vi "WDF file reader for YokaogawaDL850.vi"() -> ()   [LabVIEW 2010]
uses:
  <vilib>/Platform/storage/lvStorage.llb/xStorage/Open Data Storage/Open Data Storage.xnode
  <vilib>/Platform/storage/lvStorage.llb/_openFunction.ctl
  <vilib>/Platform/storage/lvStorage.llb/xStorage/Read Data/Read Data.xnode
  <vilib>/Platform/storage/lvStorage.llb/xStorage/Close Data Storage/Close Data Storage.xnode
  <vilib>/Analysis/3filter.llb/Filter Passband Type.ctl
  <vilib>/Platform/storage/lvStorage.llb/_openStorageWithRootAutoDetect.vi
  <vilib>/Platform/storage/lvStorage.llb/xStorage/xStorageSupp/ErrorOut.vi
  <vilib>/Platform/storage/lvStorage.llb/_queryPropDateTime.vi
  <vilib>/Platform/storage/lvStorage.llb/_queryGenericObjects.vi
  <vilib>/Platform/storage/lvStorage.llb/_loadAllDouble.vi
  <vilib>/Platform/storage/Storage.llb/Get Object Info.vi
  <vilib>/Platform/storage/Storage.llb/__closeStorageFromObject.vi
  <vilib>/Analysis/3filter.llb/Butterworth Filter (DBL).vi
  <vilib>/measure/maspectr.llb/FFT Power Spectrum and PSD for 1 Chan.vi
  <vilib>/Analysis/2dsp.llb/1D Auto Correlation (DBL).vi
  <vilib>/Analysis/2dsp.llb/1D Cross Correlation (DBL).vi
  <vilib>/Utility/file.llb/Write To Spreadsheet File (DBL).vi
  <vilib>/Utility/file.llb/Write To Spreadsheet File (string).vi
  <vilib>/measure/NI_MAPro.lvlib
  <vilib>/Analysis/NI_AALBase.lvlib
  <vilib>/Analysis/NI_AALPro.lvlib
panel:
  out "cross corr":dbl[](graph) caption="Rxx"
  in  "Check correlation":bool
  out "auto corr V":dbl[](graph) caption="Rxx"
  out "Rxx":dbl[](graph)
  in  "voltage Zero mean":bool
  in  "current Zero mean":bool
  out "saved selected data file name":string
  out "Moving average time":dbl
  in  "Moving average Window size":i32
  in  "Trace type":enum16{"current", "voltage"}(ring)
  in  "Check noise spectrum":bool
  out "Power spectrum":cluster{dbl[], "magnitude":dbl[]}(graph)
  out "Sampling rate (Hz)":dbl
  out "current trace":cluster{dbl[], "Data":dbl[]}(graph)
  in  "Save selected Data":bool
  in  "File type":string(combo)="*.wdf"
  in  "Save Data":bool
  in  "Voltage amplifier gain":dbl=10.0
  in  "Applied voltage(V)":dbl=0.1
  in  "Sampling interval (ms)":dbl=0.02
  out "CH-all":dbl[][](graph)
  out "Total data points":i32
  out "File Path":path=path "C:/JinHe/data/CNT measurement/20080324_SWCNT bundle/2MKCl1p2V5E40.txt"
  in  "Current No 2":u16
  in  "Forward":bool
  in  "back":bool
  in  "Change folder":bool
  in  "Current No":u16
  out "Total":dbl
  out "Status":string
  out "Numeric":i32
  in  "stop":bool
  out "error out":errorcluster
  out "Voltage trace":cluster{dbl[], "Array":dbl[]}[](graph)
  # "YOKOGAWA DL850 WDF file reader"
  # "Viewing files"
  # "(ms)"
  # "(points)"
  # "try save in TDMS format\nselect different noise removing function"
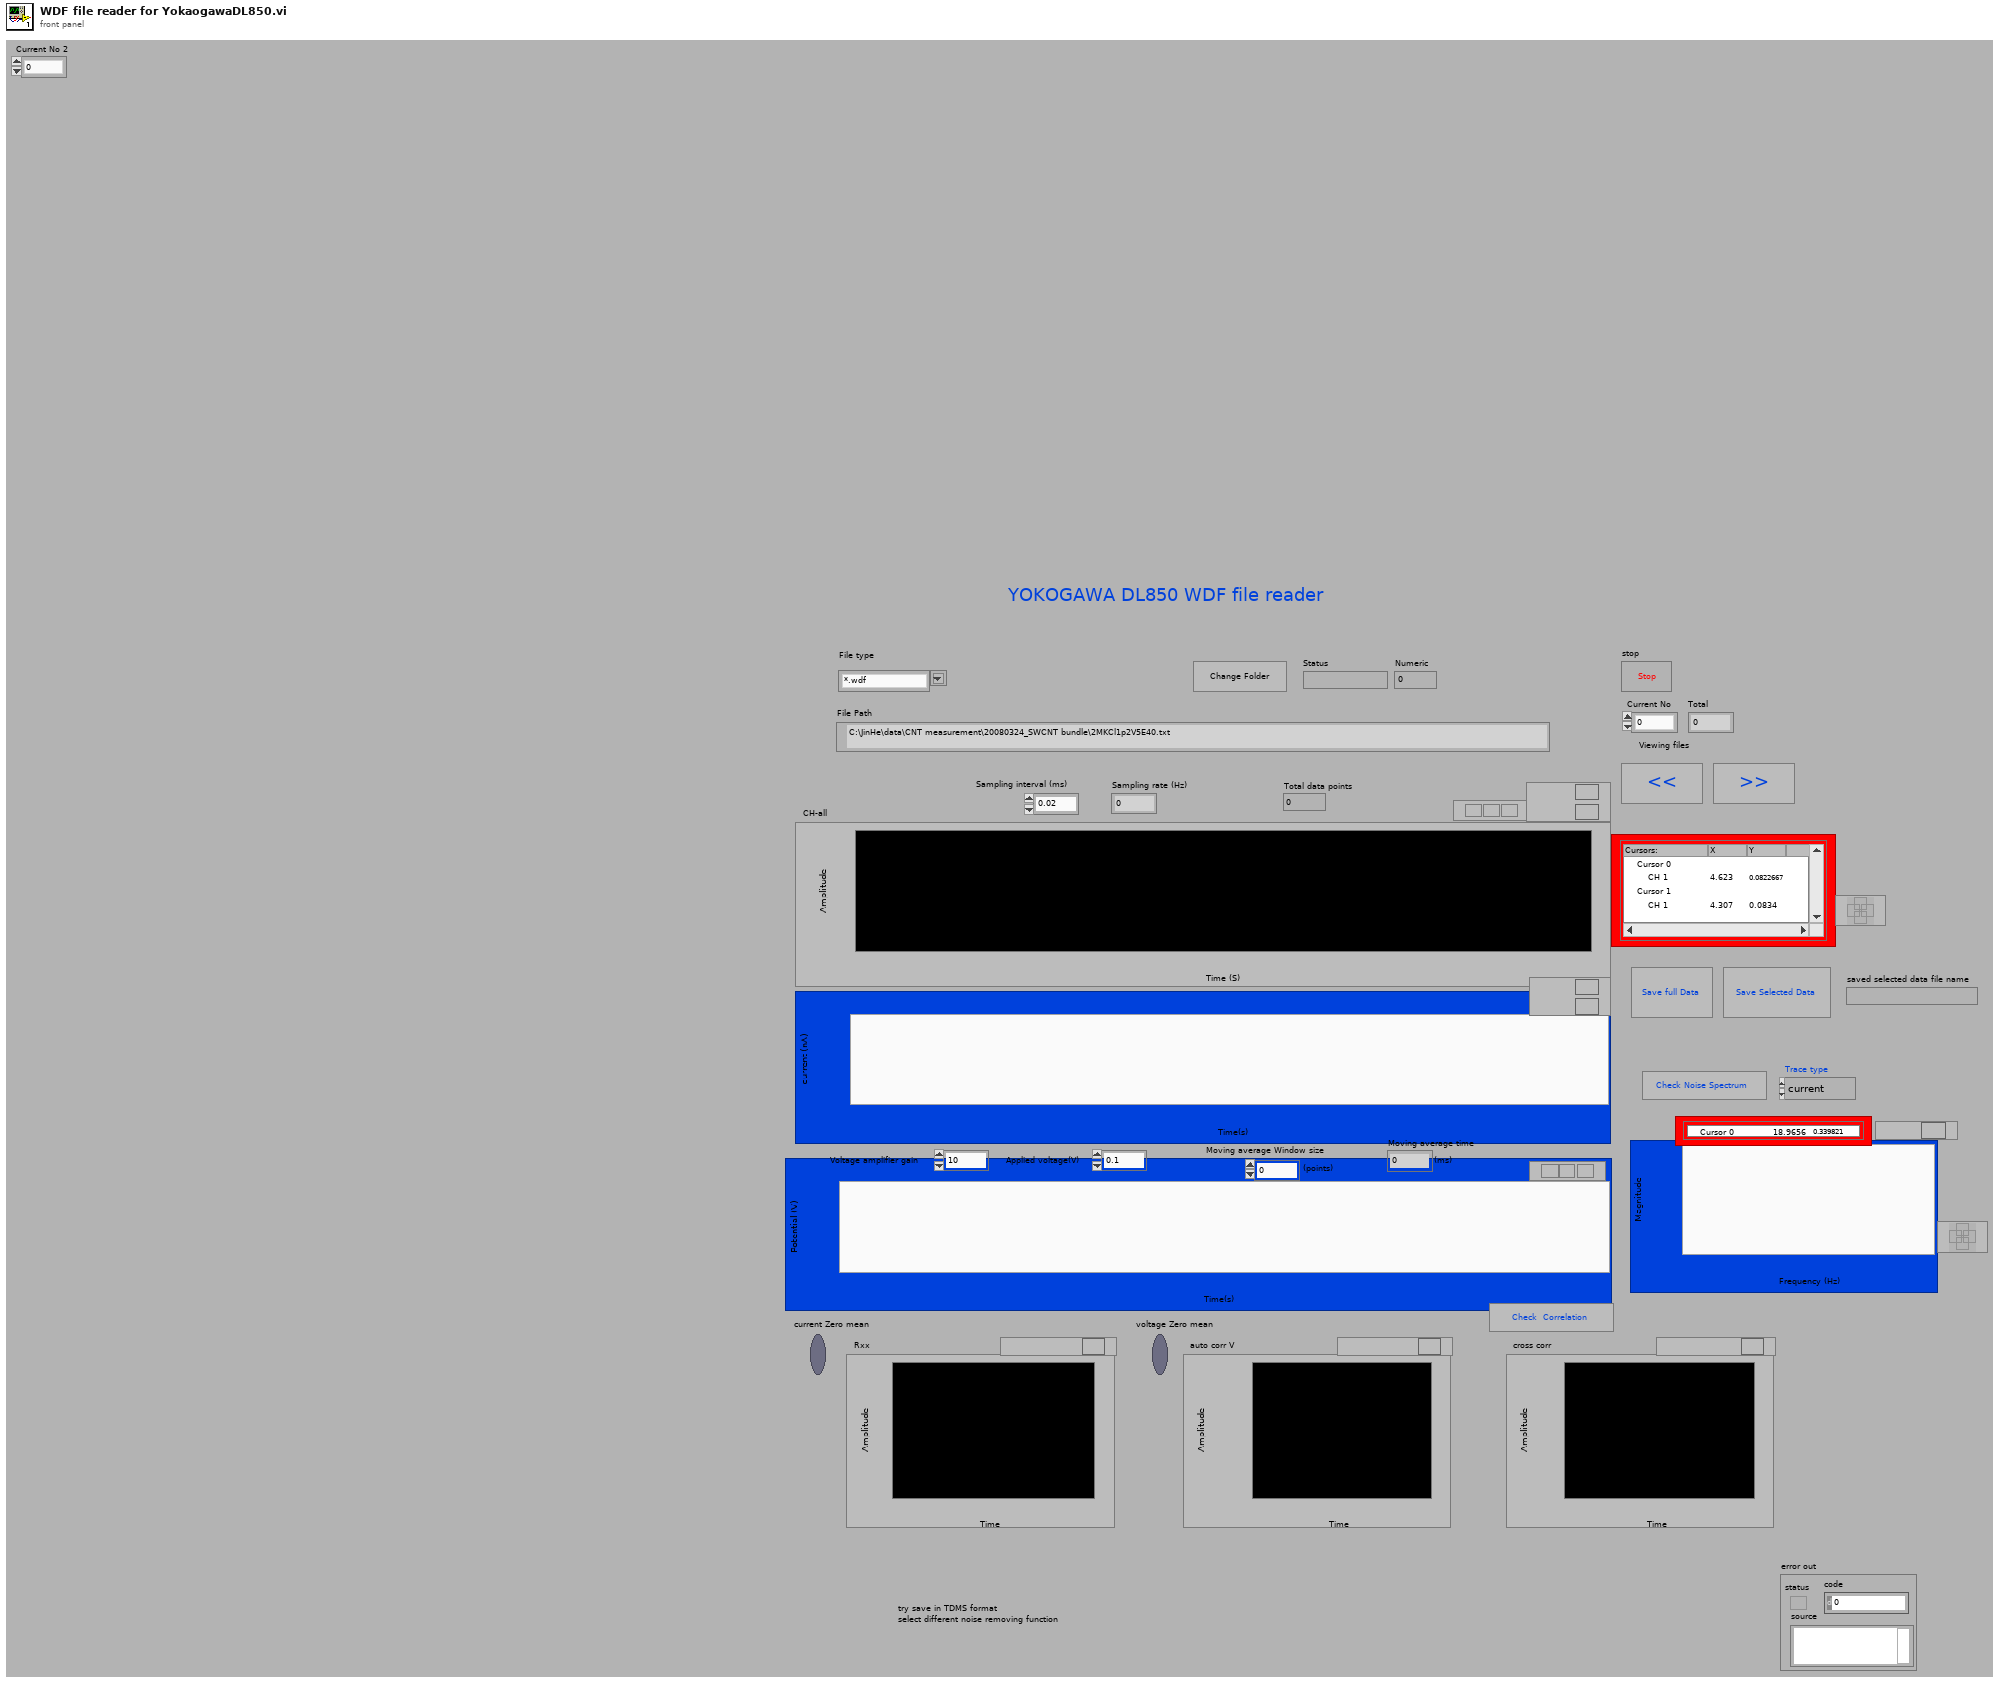
[diagram p1: front panel]
types:
  T1 = cluster{bool, "DIR path":path, "File names":string[], "File total number":i32, "File number counter":i32, "Data":dbl[][], "offset":dbl, "Peaks":dbl[][], "Step":dbl, "High":dbl, "Low":dbl, "Start":dbl, "End":dbl, "timestep(s)":dbl, "Modified Data ":dbl[][], "voltage gain":dbl, "Baseline":dbl[], "Magnitude":dbl[][], "Applied voltage (V)":dbl, "Data number":i32, "current data":dbl[][], "voltage data":dbl[][], "File type":string, "Cursor X1":dbl, "Cursor X0":dbl, "Time":dbl[], "Selected data":dbl[][]}
  T2 = enum16{"UPDATE", "READ", "QUERY", "CREATE CHILD", "CREATE", "CONNECT", "DISCONNECT"}
  T3 = typedef "_openFunction.ctl" = enum16{"open", "open or create", "create or replace", "create", "open (read only)"}
  T4 = typedef "NI_AALBase.lvlib/Filter Passband Type.ctl" = enum32{"Lowpass", "Highpass", "Bandpass", "Bandstop"}
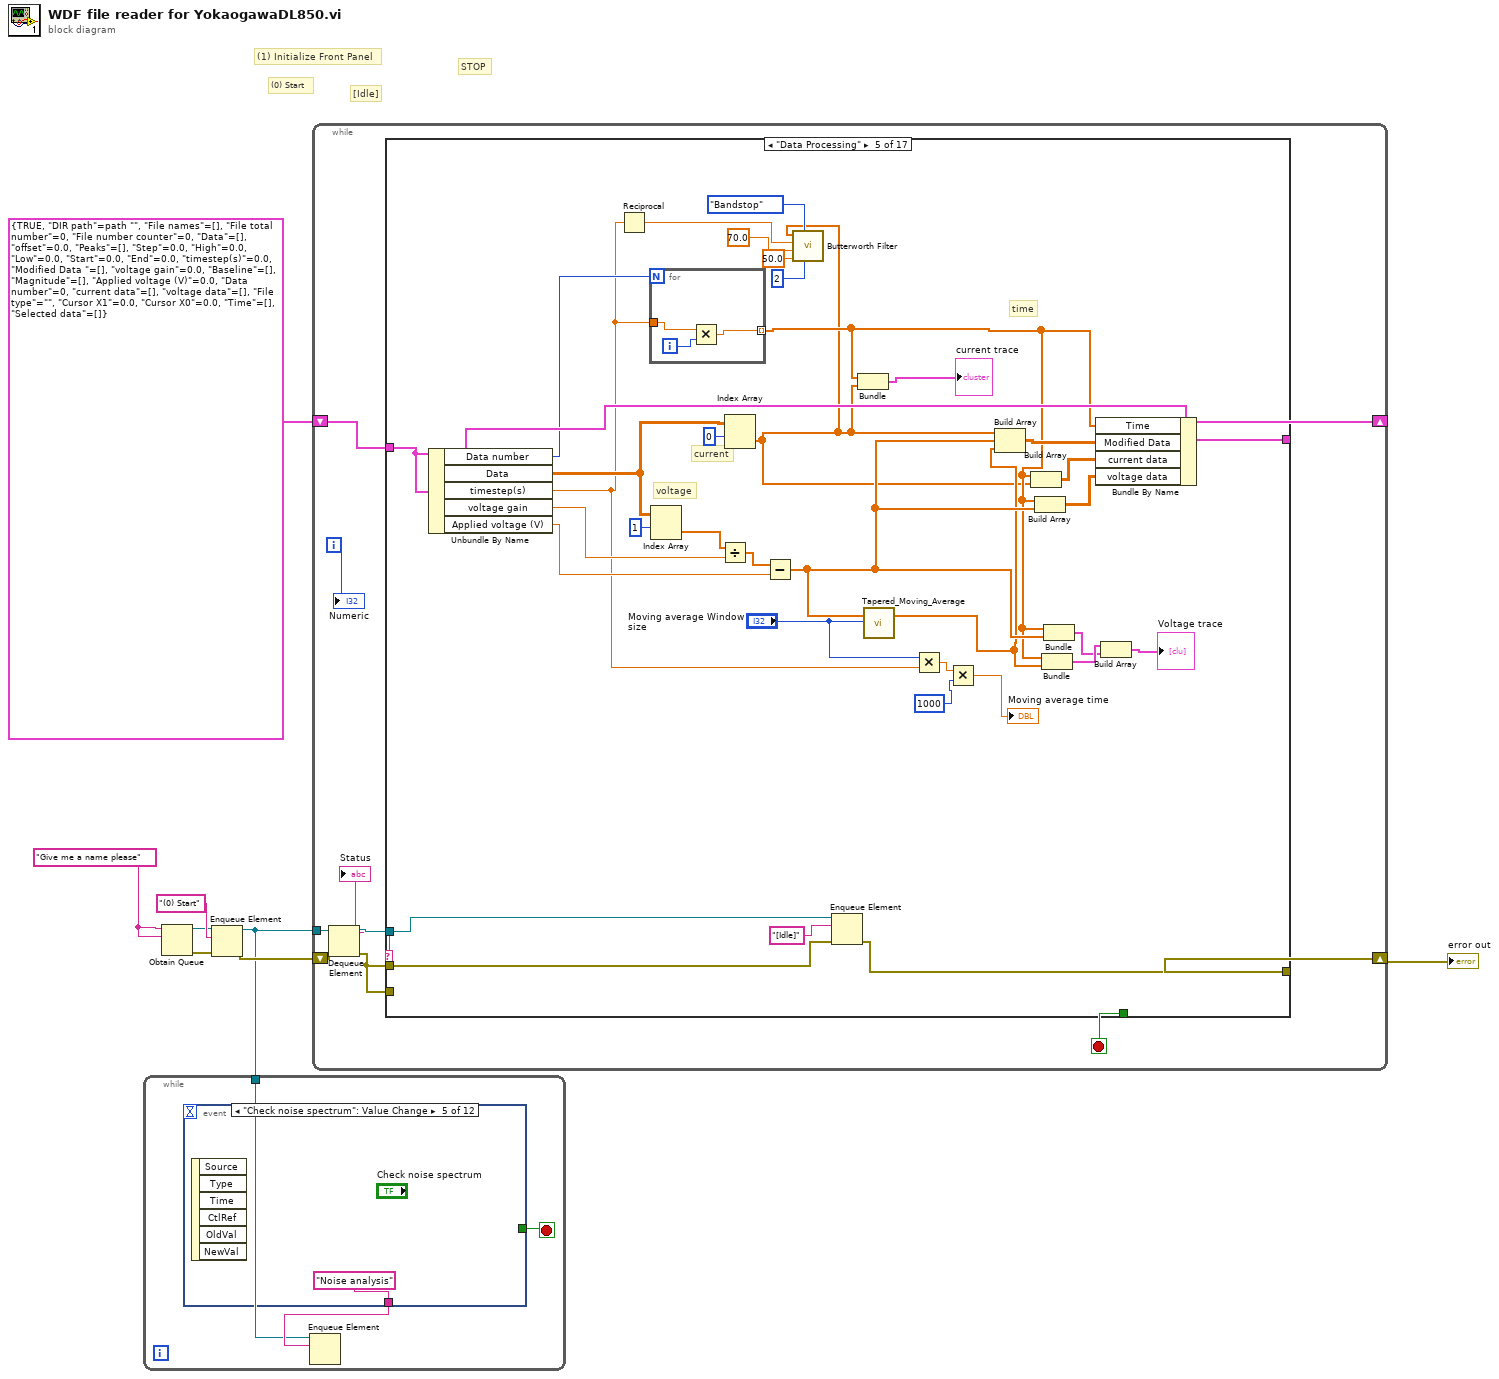
[diagram p0: block diagram]
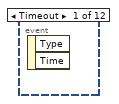
[diagram p2: hidden frame]
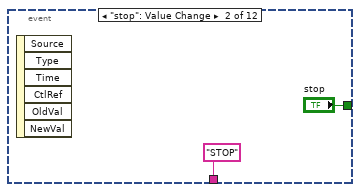
[diagram p3: hidden frame]
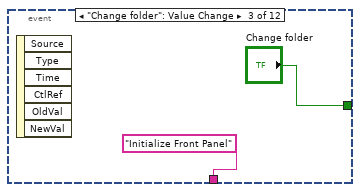
[diagram p4: hidden frame]
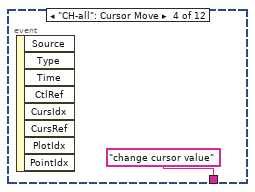
[diagram p5: hidden frame]
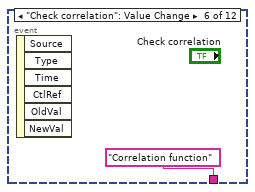
[diagram p6: hidden frame]
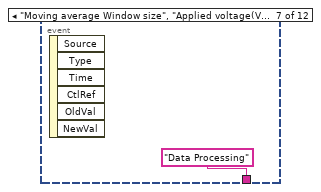
[diagram p7: hidden frame]
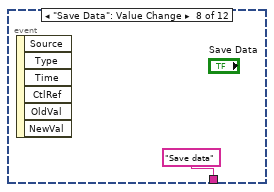
[diagram p8: hidden frame]
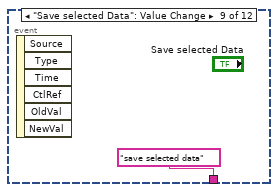
[diagram p9: hidden frame]
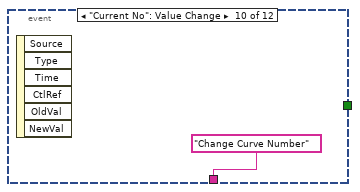
[diagram p10: hidden frame]
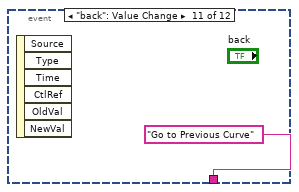
[diagram p11: hidden frame]
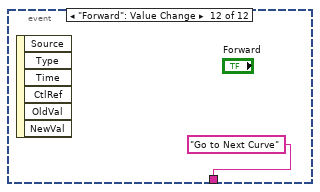
[diagram p12: hidden frame]
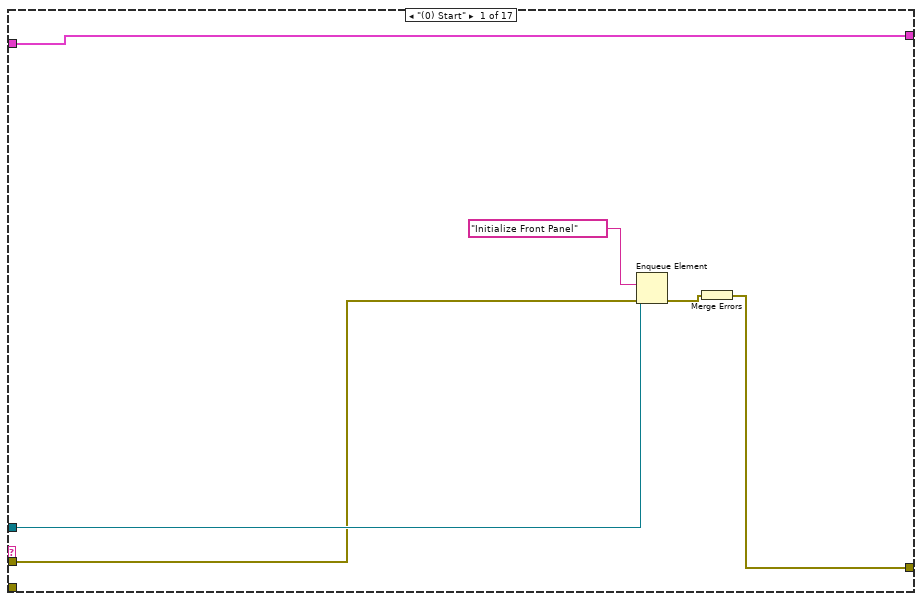
[diagram p13: hidden frame]
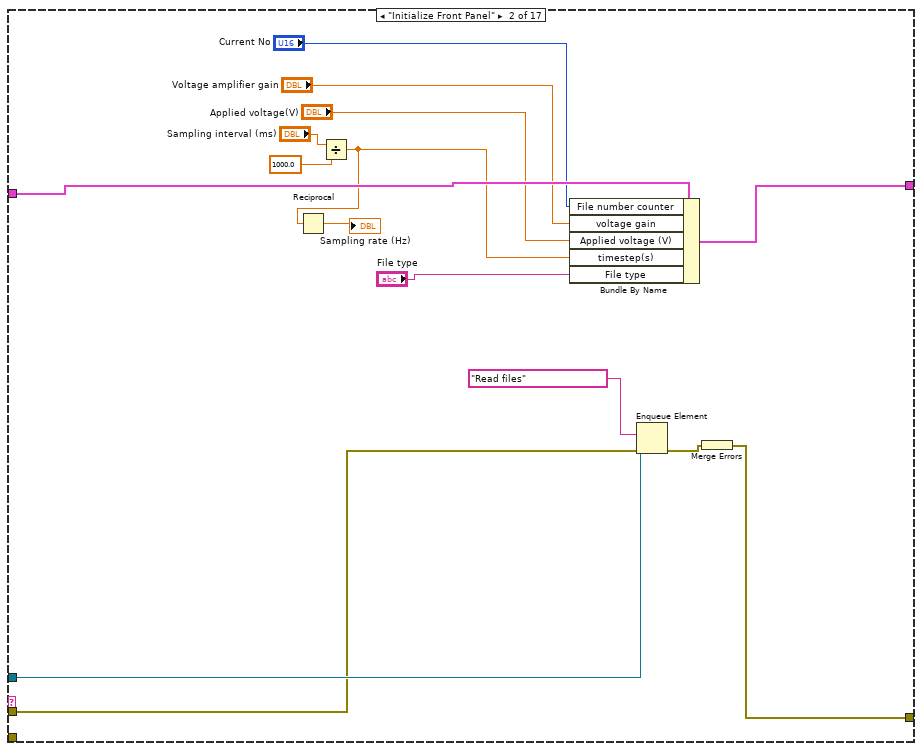
[diagram p14: hidden frame]
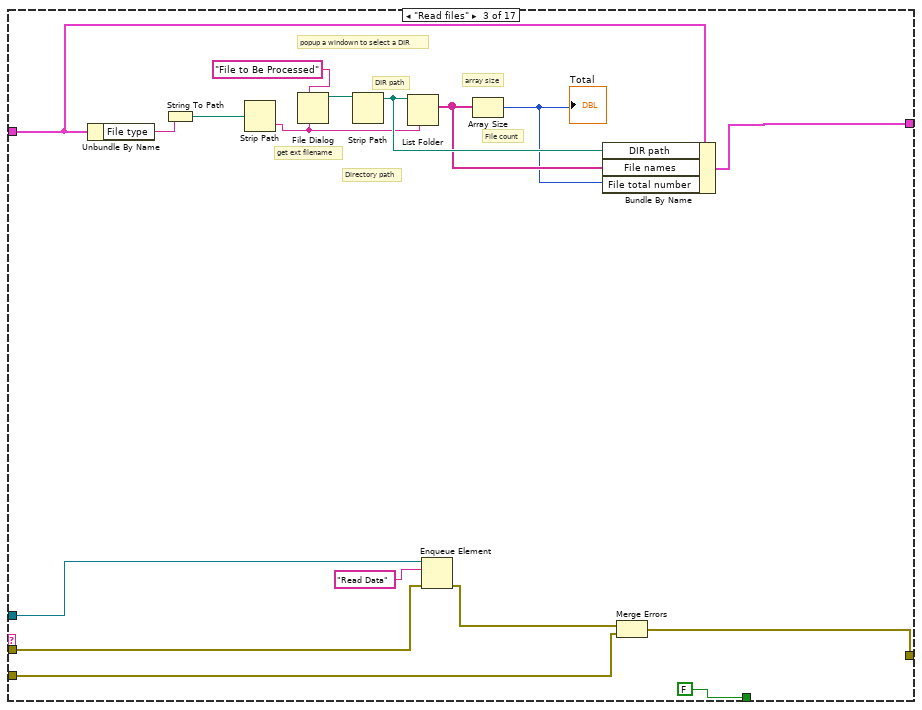
[diagram p15: hidden frame]
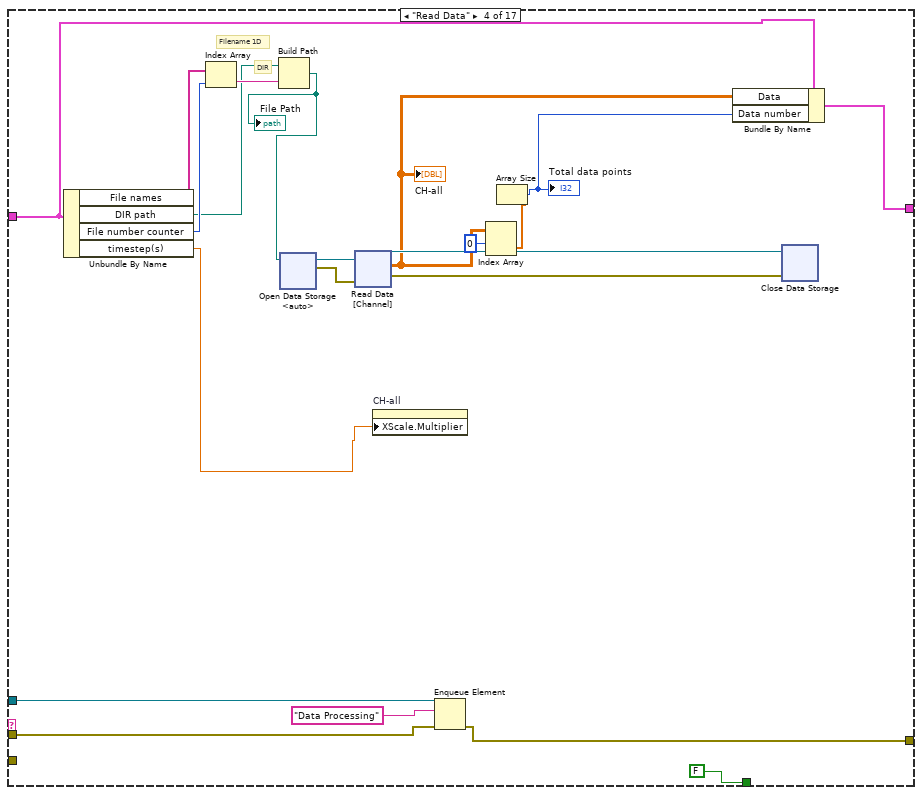
[diagram p16: hidden frame]
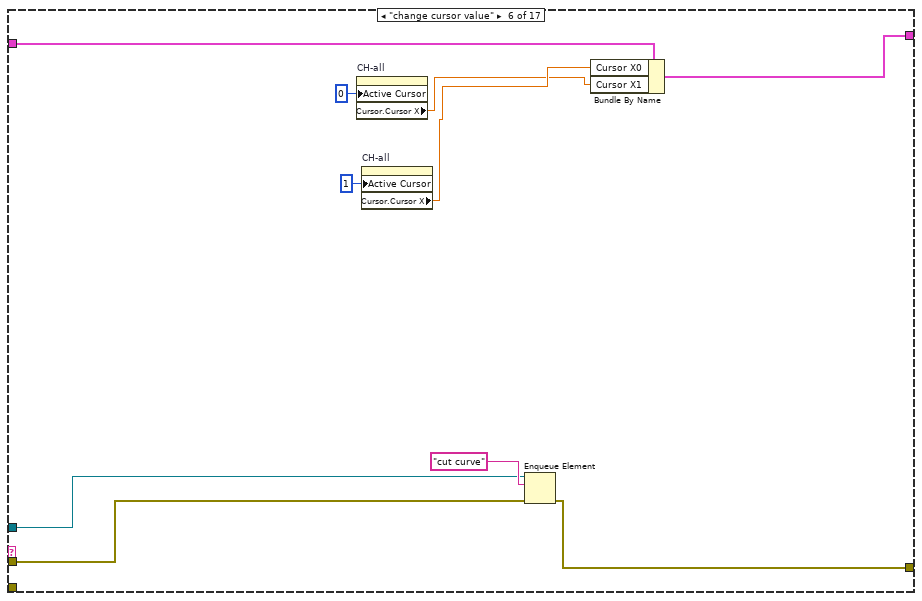
[diagram p17: hidden frame]
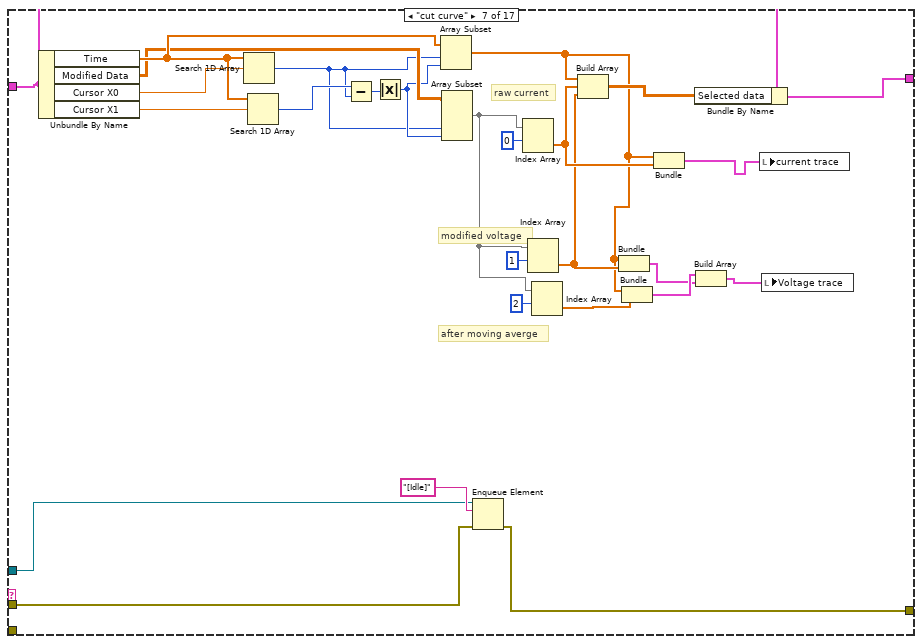
[diagram p18: hidden frame]
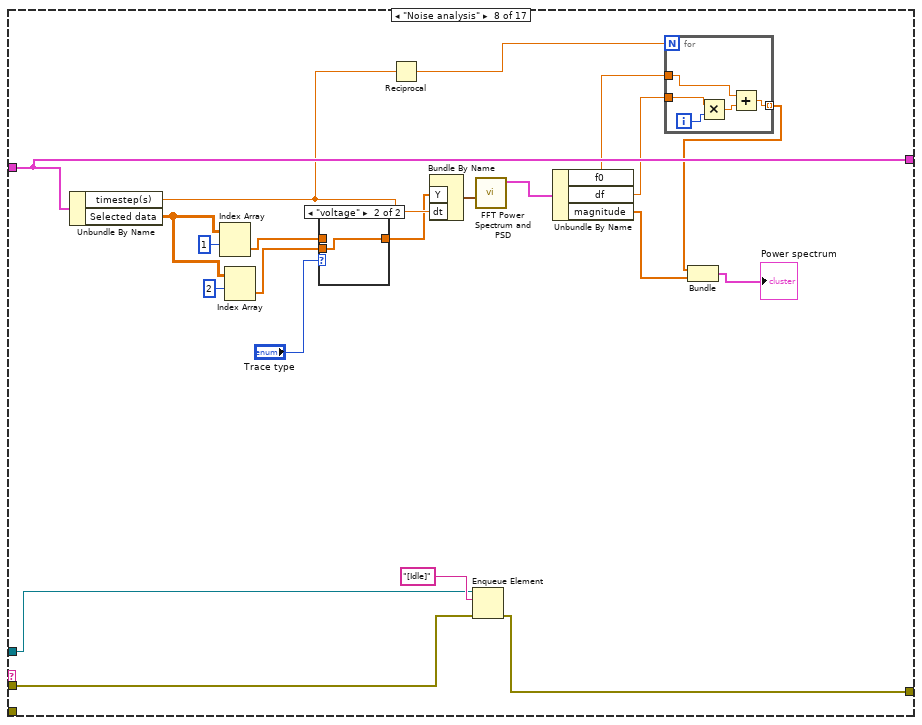
[diagram p19: hidden frame]
diagram:
  w1 = "Give me a name please" ("name (unnamed)")
  # "STOP"
  # "[Idle]"
  # "(1) Initialize Front Panel"
  # "(0) Start"
  n1 = Obtain Queue(name (unnamed)=w1, element data type=w1) -> (queue out=w3:refnum<queue>, error out=w2:errorcluster)  [unwired: 3 in, 1 out]
  n2 = Enqueue Element(queue=w3, element="(0) Start", error in (no error)=w2) -> (queue out=w5:refnum<queue>, error out=w7:errorcluster)  [unwired: 2 out]
  n3 = while {
    tunnel: w5 -> [w9]
    stop <- w11 stop-if-true
    n4 = event shown="[4] \"Check noise spectrum\": Value Change" {
      selector: _ -> [_ _ _ _ _ _ _ _ _ _ _ _]
      dyn-events: _ -> [_ _ _ _ _ _ _ _ _ _ _ _]
      timeout: _ -> [_ _ _ _ _ _ _ _ _ _ _ _]
      tunnel: [_ "stop" "Change folder" _ _ _ _ _ _ _ _ _] -> w11
      tunnel: [_ "STOP" ("element") "Initialize Front Panel" ("element") "change cursor value" ("element") "Noise analysis" ("element") "Correlation function" ("element") "Data Processing" ("element") "Save data" ("element") "save selected data" ("element") "Change Curve Number" "Go to Previous Curve" "Go to Next Curve"] -> w10
      event Timeout {
        n5 = event-data() -> ()  [unwired: 3 out]
      }
      event "stop": Value Change {
        n6 = event-data() -> ()  [unwired: 7 out]
      }
      event "Change folder": Value Change {
        n7 = event-data() -> ()  [unwired: 7 out]
      }
      event "CH-all": Cursor Move {
        n8 = event-data() -> ()  [unwired: 9 out]
      }
      event "Check noise spectrum": Value Change {
        n9 = event-data() -> ()  [unwired: 7 out]
      }
      event "Check correlation": Value Change {
        n10 = event-data() -> ()  [unwired: 7 out]
      }
      event "Moving average Window size", "Applied voltage(V)", "Voltage amplifier gain", "Sampling interval (ms)": Value Change {
        n11 = event-data() -> ()  [unwired: 7 out]
      }
      event "Save Data": Value Change {
        n12 = event-data() -> ()  [unwired: 7 out]
      }
      event "Save selected Data": Value Change {
        n13 = event-data() -> ()  [unwired: 7 out]
      }
      event "Current No": Value Change {
        n14 = event-data() -> ()  [unwired: 7 out]
      }
      event "back": Value Change {
        n15 = event-data() -> ()  [unwired: 7 out]
      }
      event "Forward": Value Change {
        n16 = event-data() -> ()  [unwired: 7 out]
      }
    }
    n17 = Enqueue Element(queue=w9, element=w10) -> ()  [unwired: 1 in, 4 out]
  }
  n18 = while {
    shift-right: [w31] -> w6
    shift-left: w7 -> [w34]
    shift-right: [w25] -> _
    shift-left: T1 {TRUE, "DIR path"=path "", "File names"=[], "File total number"=0, "File number counter"=0, "Data"=[], "offset"=0.0, "Peaks"=[], "Step"=0.0, "High"=0.0, "Low"=0.0, "Start"=0.0, "End"=0.0, "timestep(s)"=0.0, "Modified Data "=[], "voltage gain"=0.0, "Baseline"=[], "Magnitude"=[], "Applied voltage (V)"=0.0, "Data number"=0, "current data"=[], "voltage data"=[], "File type"="", "Cursor X1"=0.0, "Cursor X0"=0.0, "Time"=[], "Selected data"=[]} -> [w26]
    tunnel: w5 -> [w30]
    i -> [w27]
    stop <- w28 stop-if-true
    n19 = Dequeue Element(queue=w30, error in (no error)=w34) -> (queue out=w33:refnum<queue>, element=w32:string, error out=w29:errorcluster)  [unwired: 2 out]
    "Status" <- w32
    n20 = case shown="\"Data Processing\"" w32 {
      tunnel: w33 -> [w40 w55 w66 w91 w152 w170 w192 w215 w256 w294 w310 w328 w345 w362 w373 _ w384]
      tunnel: w29 -> [w38 w53 w63 w89 w154 w173 w191 w217 w258 w296 w312 _ _ _ w370 w377 w383]
      tunnel: [w36 w51 w65 w90 w153 w172 w190 w216 w257 w295 w311 w326 w343 w363 w374 w376 w381] -> w31
      tunnel: w29 -> [_ _ w62 _ _ _ _ _ _ _ _ w327 w344 w364 _ _ _]
      tunnel: [_ _ FALSE FALSE _ _ _ _ _ _ _ FALSE FALSE _ TRUE _ _] -> w28
      tunnel: w26 -> [w35 w50 w58 w77 w157 w175 w201 w223 w263 w293 w309 w331 w349 w360 w366 w375 w378]
      tunnel: [w35 w49 w71 w76 w156 w174 w202 w223 w263 w293 w309 w330 w348 w359 w366 w375 w378] -> w25
      frame "(0) Start" {
        n21 = Enqueue Element(queue=w40, element="Initialize Front Panel", error in (no error)=w38) -> (error out=w37:errorcluster)  [unwired: 3 out]
        n22 = Merge Errors(w37) -> (w36:errorcluster)
      }
      frame "Initialize Front Panel" {
        n23 = Divide(x="Sampling interval (ms)", y=1000.0) -> (x/y=w41:dbl)
        n24 = Reciprocal(x=w41) -> (1/x=→"Sampling rate (Hz)":dbl)
        n25 = Bundle By Name(cluster=w50, "File number counter"="Current No", "voltage gain"="Voltage amplifier gain", "Applied voltage (V)"="Applied voltage(V)", "timestep(s)"=w41, "File type"="File type") -> (w49:T1)
        n26 = Enqueue Element(queue=w55, element="Read files", error in (no error)=w53) -> (error out=w52:errorcluster)  [unwired: 3 out]
        n27 = Merge Errors(w52) -> (w51:errorcluster)
      }
      frame "Read files" {
        # "DIR path"
        # "File count"
        # "popup a windown to select a DIR"
        # "get ext filename"
        # "Directory path"
        # "array size"
        n28 = Unbundle By Name(w58) -> ("File type"=w57:string)
        n29 = String To Path(string=w57) -> (path=w56:path)
        n30 = Strip Path(path=w56) -> (name=w59:string)  [unwired: 1 out]
        n31 = File Dialog(6:w59, 7:"File to Be Processed") -> (3:w72:path)  [unwired: 1 in, 7 out]
        n32 = Strip Path(path=w72) -> (stripped path=w70:path)  [unwired: 1 out]
        n33 = List Folder(path=w70, pattern=w59) -> (filenames=w69:string[])  [unwired: 1 in, 4 out]
        n34 = Enqueue Element(queue=w66, element="Read Data", error in (no error)=w63) -> (error out=w64:errorcluster)  [unwired: 3 out]
        n35 = Array Size(array=w69) -> (size(s)=w68:i32)
        "Total" <- w68
        n36 = Bundle By Name(cluster=w58, "DIR path"=w70, "File names"=w69, "File total number"=w68) -> (w71:T1)
        n37 = Merge Errors(w64, w62) -> (w65:errorcluster)
      }
      frame "Read Data" {
        # "DIR"
        # "Filename 1D"
        n38 = Unbundle By Name(w77) -> ("File names"=w87:string[], "DIR path"=w85:path, "File number counter"=w86:i32, "timestep(s)"=w74:dbl)
        n39 = Index Array(array=w87, index=w86) -> (element=w88:string)
        n40 = Build Path(base path=w85, name or relative path=w88) -> (appended path=w84:path)
        "File Path" <- w84
        n41 = xnode "Open Data Storage\n<auto>"("file path"=w84) -> ("storage refnum (file)"=w83:refnum<k20>, "error out"=w82:errorcluster)  [unwired: 4 in, 1 out]
        n42 = xnode "Read Data\n[Channel]"("storage refnum (file)"=w83, "error in"=w82) -> ("storage refnum (file) out"=w80:refnum<k20>, "error out"=w81:errorcluster, "Signal"=w75:dbl[][])  [unwired: 2 in, 1 out]
        "CH-all" <- w75
        n43 = property on="CH-all" class="WFGraph (strict)"("XScale.Multiplier"=w74) -> ()  [unwired: 2 in, 2 out]
        n44 = Enqueue Element(queue=w91, element="Data Processing", error in (no error)=w89) -> (error out=w90:errorcluster)  [unwired: 3 out]
        n45 = Index Array(array=w75, index (row)=0) -> (element=w78:dbl[])  [unwired: 1 in]
        n46 = Array Size(array=w78) -> (size(s)=w73:i32)
        "Total data points" <- w73
        n47 = Bundle By Name(cluster=w77, "Data"=w75, "Data number"=w73) -> (w76:T1)
        n48 = xnode "Close Data Storage"("storage refnum (file)"=w80, "error in (no error)"=w81) -> ()  [unwired: 2 out]
      }
      frame "Data Processing" {
        # "time"
        # "voltage"
        # "current"
        n49 = Unbundle By Name(w157) -> ("Data number"=w148:i32, "Data"=w158:dbl[][], "timestep(s)"=w134:dbl, "voltage gain"=w151:dbl, "Applied voltage (V)"=w150:dbl)
        n50 = Reciprocal(x=w134) -> (1/x=w133:dbl)
        n51 = for {
          N: w148 -> [_]
          tunnel: w134 -> [w164]
          tunnel: [w163] -> w130 mode=indexing
          i -> [w165]
          n52 = Multiply(x=w164, y=w165) -> (x*y=w163:dbl)
        }
        n53 = Index Array(array=w158, index (row)=1) -> (element=w161:dbl[])  [unwired: 1 in]
        n54 = Divide(x=w161, y=w151) -> (x/y=w160:dbl[])
        n55 = Index Array(array=w158, index (row)=0) -> (element=w129:dbl[])  [unwired: 1 in]
        n56 = Subtract(x=w160, y=w150) -> (x-y=w142:dbl[])
        n57 = call-poly <vilib>:"Butterworth Filter.vi"("order"=2, "filter type"=Filter_Passband_Type."Bandstop", "low cutoff freq: fl"=50.0, "high cutoff freq: fh"=70.0 ("sampling freq: fs"), "sampling freq: fs"=w133, "X"=w129) -> ()  [unwired: 2 in, 2 out]
        n58 = Enqueue Element(queue=w152, element="[Idle]", error in (no error)=w154) -> (error out=w153:errorcluster)  [unwired: 3 out]
        n59 = Bundle(w130, "Data"=w129) -> (→"current trace":cluster{dbl[], "Data":dbl[]})  [unwired: 1 out]
        n60 = call "Tapered_Moving_Average.vi"("Data to be averaged"=w142, "Window size"="Moving average Window size") -> ("Averaged data"=w141:dbl[])  [unwired: 17 in]
        n61 = Multiply(x="Moving average Window size", y=w134) -> (x*y=w140:dbl)
        n62 = Multiply(x=w140, y=1000 ("index (row)")) -> (x*y=→"Moving average time":dbl)
        n63 = Build Array(w129, w142, w141) -> (w149:dbl[][])
        n64 = Build Array(w130, w129) -> (w147:dbl[][])
        n65 = Build Array(w130, w142) -> (w146:dbl[][])
        n66 = Bundle(w130, "Averaged data"=w141) -> (w144:cluster{dbl[], "Averaged data":dbl[]})  [unwired: 1 out]
        n67 = Bundle(w130, w142) -> (w143:cluster{dbl[], dbl[]})  [unwired: 1 out]
        n68 = Bundle By Name(cluster=w157, "Time"=w130, "Modified Data"=w149, "current data"=w147, "voltage data"=w146) -> (w156:T1)
        n69 = Build Array(w144, w143) -> (→"Voltage trace":cluster{dbl[], "Averaged data":dbl[]}[])
      }
      frame "change cursor value" {
        n70 = property on="CH-all" class="WFGraph (strict)"("Active Cursor"=u32 0) -> ("Cursor.Cursor X"=w166:dbl)  [unwired: 2 in, 2 out]
        n71 = property on="CH-all" class="WFGraph (strict)"("Active Cursor"=u32 1) -> ("Cursor.Cursor X"=w167:dbl)  [unwired: 2 in, 2 out]
        n72 = Enqueue Element(queue=w170, element="cut curve", error in (no error)=w173) -> (error out=w172:errorcluster)  [unwired: 1 in, 2 out]
        n73 = Bundle By Name(cluster=w175, "Cursor X0"=w167, "Cursor X1"=w166) -> (w174:T1)
      }
      frame "cut curve" {
        # "after moving averge"
        # "modified voltage"
        # "raw current"
        n74 = Unbundle By Name(w201) -> ("Time"=w198:dbl[], "Modified Data"=w195:dbl[][], "Cursor X0"=w196:dbl, "Cursor X1"=w197:dbl)
        n75 = Search 1D Array(1D array=w198, element=w196) -> (index of element=w186:i32)  [unwired: 1 in]
        n76 = Search 1D Array(1D array=w198, element=w197) -> (index of element=w200:i32)  [unwired: 1 in]
        n77 = Subtract(x=w200, y=w186) -> (x-y=w199:i32)
        n78 = Absolute Value(x=w199) -> (abs(x)=w187:i32)
        n79 = Array Subset(array=w198, index=w186, length=w187) -> (w177:dbl[])
        n80 = Array Subset(array=w195, index (col)=w186, length (col)=w187) -> (w178:dbl[][])  [unwired: 2 in]
        n81 = Enqueue Element(queue=w192, element="[Idle]", error in (no error)=w191) -> (error out=w190:errorcluster)  [unwired: 1 in, 2 out]
        n82 = Index Array(array=w178, index (row)=0) -> (element=w185:dbl[])  [unwired: 1 in]
        n83 = Index Array(array=w178, index (row)=1) -> (element=w184:dbl[])  [unwired: 1 in]
        n84 = Index Array(array=w178, index (row)=2) -> (element=w182:dbl[])  [unwired: 1 in]
        n85 = Build Array(w177, w185, w184) -> (w194:dbl[][])
        n86 = Bundle(w177, w184) -> (w180:cluster{dbl[], dbl[]})  [unwired: 1 out]
        n87 = Bundle(w177, w182) -> (w181:cluster{dbl[], dbl[]})  [unwired: 1 out]
        n88 = Bundle(w177, w185) -> (w176:cluster{dbl[], dbl[]})  [unwired: 1 out]
        n89 = Bundle By Name(cluster=w201, "Selected data"=w194) -> (w202:T1)
        n90 = Build Array(w181, w180) -> (w179:cluster{dbl[], dbl[]}[])
        n91 = local write "current trace"(w176) -> ()
        n92 = local write "Voltage trace"(w179) -> ()
      }
      frame "Noise analysis" {
        n93 = Unbundle By Name(w223) -> ("timestep(s)"=w209:dbl, "Selected data"=w220:dbl[][])
        n94 = Index Array(array=w220, index (row)=1) -> (element=w205:dbl[])  [unwired: 1 in]
        n95 = Index Array(array=w220, index (row)=2) -> (element=w204:dbl[])  [unwired: 1 in]
        n96 = case shown="\"voltage\"" "Trace type" {
          tunnel: w205 -> [w224 _]
          tunnel: [w224 w225] -> w203
          tunnel: w204 -> [_ w225]
          frame "current", Default {
          }
          frame "voltage" {
          }
        }
        n97 = Reciprocal(x=w209) -> (1/x=w208:dbl)
        n98 = Bundle By Name("Y"=w203, "dt"=w209) -> (w219:waveform(dbl))  [unwired: 1 in]
        n99 = Enqueue Element(queue=w215, element="[Idle]", error in (no error)=w217) -> (error out=w216:errorcluster)  [unwired: 1 in, 2 out]
        n100 = call-poly <vilib>:"FFT Power Spectrum and PSD.vi"("time signal"=w219) -> ("Power Spectrum / PSD"=w214:cluster{"f0":dbl, "df":dbl, "magnitude":dbl[]})  [unwired: 7 in, 3 out]
        n101 = Unbundle By Name(w214) -> ("f0"=w207:dbl, "df"=w213:dbl, "magnitude"=w212:dbl[])
        n102 = for {
          N: w208 -> [_]
          tunnel: w213 -> [w229]
          tunnel: [w227] -> w211 mode=indexing
          tunnel: w207 -> [w226]
          i -> [w230]
          n103 = Multiply(x=w229, y=w230) -> (x*y=w228:dbl)
          n104 = Add(x=w226, y=w228) -> (x+y=w227:dbl)
        }
        n105 = Bundle(w211, "magnitude"=w212) -> (→"Power spectrum":cluster{dbl[], "magnitude":dbl[]})  [unwired: 1 out]
      }
      frame "Correlation function" {
        n106 = Unbundle By Name(w263) -> ("timestep(s)"=w235:dbl, "Selected data"=w260:dbl[][])
        n107 = Index Array(array=w260, index (row)=1) -> (element=w252:dbl[])  [unwired: 1 in]
        n108 = Index Array(array=w260, index (row)=2) -> (element=w241:dbl[])  [unwired: 1 in]
        n109 = Multiply(x=w241, y=1000) -> (x*y=w239:dbl[])
        n110 = call <vilib>:"Mean.vi"("X"=w252) -> ("mean"=w251:dbl)  [unwired: 1 out]
        n111 = call <vilib>:"Mean.vi"("X"=w239) -> ("mean"=w254:dbl)  [unwired: 1 out]
        n112 = Subtract(x=w252, y=w251) -> (x-y=w243:dbl[])
        n113 = Subtract(x=w239, y=w254) -> (x-y=w237:dbl[])
        n114 = Divide(x=w237, y=1000.0) -> (x/y=w236:dbl[])
        n115 = Select(t=w243, s="current Zero mean", f=w252) -> (s? t:f=w249:dbl[])
        n116 = Select(t=w236, s="voltage Zero mean", f=w241) -> (s? t:f=w253:dbl[])
        n117 = Enqueue Element(queue=w256, element="[Idle]", error in (no error)=w258) -> (error out=w257:errorcluster)  [unwired: 1 in, 2 out]
        n118 = call-poly <vilib>:"AutoCorrelation.vi"("X"=w253) -> ("Rxx"=→"auto corr V":dbl[])  [unwired: 9 in, 1 out]
        n119 = call-poly <vilib>:"AutoCorrelation.vi"("X"=w249) -> ("Rxx"=w247:dbl[])  [unwired: 9 in, 1 out]
        "Rxx" <- w247
        n120 = call-poly <vilib>:"CrossCorrelation.vi"("normalization"=enum32{"none", "unbiased", "biased"}."none", "algorithm"=enum32{"direct", "frequency domain"}."frequency domain", "Y"=w236, "X"=w243) -> ("Rxy"=→"cross corr":dbl[])  [unwired: 6 in, 1 out]
        n121 = Array Size(array=w247) -> (size(s)=w246:i32)
        n122 = Divide(x=w246, y=-2) -> (x/y=w244:dbl)
        n123 = Multiply(x=w235, y=w244) -> (x*y=w234:dbl)
        n124 = property on="auto corr V" class="WFGraph (strict)"("XScale.Multiplier"=w235, "XScale.Offset"=w234) -> ()  [unwired: 2 in, 2 out]
        n125 = property on="Rxx" class="WFGraph (strict)"("XScale.Multiplier"=w235, "XScale.Offset"=w234) -> ()  [unwired: 2 in, 2 out]
        n126 = property on="cross corr" class="WFGraph (strict)"("XScale.Multiplier"=w235, "XScale.Offset"=w234, "XScale.RngStart"=0.0 ("X Scale.Range:Start")) -> ()  [unwired: 2 in, 2 out]
      }
      frame "Save data" {
        w268 = TRUE ("transpose? (no:F)")
        w269 = "%.6f"
        n127 = Unbundle By Name(w293) -> ("DIR path"=w272:path, "File names"=w291:string[], "File number counter"=w292:i32, "Modified Data"=w265:dbl[][], "current data"=w280:dbl[][], "voltage data"=w270:dbl[][], "Time"=w266:dbl[])
        n128 = Index Array(array=w291, index=w292) -> (element=w287:string)
        n129 = Build Array (concatenate)(w266, w265) -> (w264:dbl[][])
        n130 = Transpose 2D Array(2D array=w264) -> (transposed array=w282:dbl[][])
        n131 = Match Pattern(string=w287, regular expression=".WDF") -> (before substring=w267:string)  [unwired: 4 out]
        n132 = Enqueue Element(queue=w294, element="[Idle]", error in (no error)=w296) -> (error out=w295:errorcluster)  [unwired: 3 out]
        n133 = Concatenate Strings(w267, "changed", ".txt") -> (w286:string)
        n134 = Concatenate Strings(w267, "changedcurrent", ".txt") -> (w277:string)
        n135 = Build Path(base path=w272, name or relative path=w286) -> (appended path=w284:path)
        n136 = Concatenate Strings(w267, "changedvoltage", ".txt") -> (w273:string)
        n137 = Build Path(base path=w272, name or relative path=w277) -> (appended path=w276:path)
        n138 = Build Path(base path=w272, name or relative path=w273) -> (appended path=w271:path)
        n139 = call-poly <vilib>:"Write To Spreadsheet File.vi"("1D data"=string[] ["Time(S)", "I(nA)", "V(V)", "mov ave V", ""], "file path (dialog if empty)"=w284) -> ("new file path (Not A Path if cancelled)"=w283:path)  [unwired: 4 in, 2 out]
        n140 = call-poly <vilib>:"Write To Spreadsheet File.vi"("transpose? (no:F)"=w268, "format (%.3f)"=w269, "2D data"=w270, "file path (dialog if empty)"=w271) -> ()  [unwired: 2 in, 3 out]
        n141 = call-poly <vilib>:"Write To Spreadsheet File.vi"("transpose? (no:F)"=w268, "format (%.3f)"=w269, "2D data"=w280, "file path (dialog if empty)"=w276) -> ()  [unwired: 2 in, 3 out]
        n142 = call-poly <vilib>:"Write To Spreadsheet File.vi"("format (%.3f)"=w269, "append to file? (new file:F)"=TRUE, "2D data"=w282, "file path (dialog if empty)"=w283) -> ()  [unwired: 2 in, 3 out]
      }
      frame "save selected data" {
        n143 = Unbundle By Name(w309) -> ("DIR path"=w302:path, "File names"=w305:string[], "File number counter"=w304:i32, "Selected data"=w307:dbl[][])
        n144 = Index Array(array=w305, index=w304) -> (element=w299:string)
        n145 = List Folder(path=w302, pattern="*selected*") -> (filenames=w300:string[])  [unwired: 2 in, 3 out]
        n146 = while {
          tunnel: w300 -> [w317]
          tunnel: w299 -> [w320]
          tunnel: [w314] -> w298
          i -> [w318]
          stop <- w315 stop-if-true
          n147 = Number To Decimal String(number=w318) -> (decimal integer string=w319:string)  [unwired: 1 in]
          n148 = Match Pattern(string=w320, regular expression=".WDF") -> (before substring=w322:string)  [unwired: 4 out]
          n149 = Concatenate Strings(w322, "selected" ("string"), w319, ".txt") -> (w314:string)
          n150 = Search 1D Array(1D array=w317, element=w314) -> (index of element=w316:i32)  [unwired: 1 in]
          n151 = Less Or Equal To 0?(x=w316) -> (x <= 0?=w315:bool)
        }
        "saved selected data file name" <- w298
        n152 = Enqueue Element(queue=w310, element="[Idle]", error in (no error)=w312) -> (error out=w311:errorcluster)  [unwired: 3 out]
        n153 = Build Path(base path=w302, name or relative path=w298) -> (appended path=w303:path)
        n154 = call-poly <vilib>:"Write To Spreadsheet File.vi"("transpose? (no:F)"=TRUE, "format (%.3f)"="%.7f", "2D data"=w307, "file path (dialog if empty)"=w303) -> ()  [unwired: 2 in, 3 out]
      }
      frame "Go to Next Curve" {
        n155 = Unbundle By Name(w331) -> ("File number counter"=w332:i32, "File total number"=w333:i32)
        n156 = Equal?(x=w332, y=w333) -> (x = y?=w334:bool)
        n157 = case shown="False" w334 {
          tunnel: w332 -> [w339 _]
          tunnel: w331 -> [w338 w341]
          tunnel: [w336 w341] -> w330
          frame False {
            n158 = Increment(x=w339) -> (x+1=w337:i32)
            n159 = property on="Forward" class="Bool"("BoolText.Text"=">>") -> ()  [unwired: 2 in, 2 out]
            n160 = local write "Current No"(w337) -> ()
            n161 = Bundle By Name(cluster=w338, "File number counter"=w337) -> (w336:T1)
          }
          frame True {
            n162 = property on="Forward" class="Bool"("BoolText.Text"="||") -> ()  [unwired: 2 in, 2 out]
          }
        }
        n163 = Enqueue Element(queue=w328, element="Read Data", error in (no error)=w327) -> (error out=w326:errorcluster)  [unwired: 3 out]
      }
      frame "Go to Previous Curve" {
        n164 = Unbundle By Name(w349) -> ("File number counter"=w350:i32)  [unwired: 1 out]
        n165 = Equal?(x=w350, y=0) -> (x = y?=w351:bool)
        n166 = case shown="False" w351 {
          tunnel: w350 -> [w354 _]
          tunnel: w349 -> [w356 w358]
          tunnel: [w355 w358] -> w348
          frame False {
            n167 = Decrement(x=w354) -> (x-1=w353:i32)
            n168 = local write "Current No"(w353) -> ()
            n169 = property on="back" class="Bool"("BoolText.Text"="<<") -> ()  [unwired: 2 in, 2 out]
            n170 = Bundle By Name(cluster=w356, "File number counter"=w353) -> (w355:T1)
          }
          frame True {
            n171 = property on="back" class="Bool"("BoolText.Text"="||") -> ()  [unwired: 2 in, 2 out]
          }
        }
        n172 = Enqueue Element(queue=w345, element="Read Data", error in (no error)=w344) -> (error out=w343:errorcluster)  [unwired: 3 out]
      }
      frame "Change Curve Number" {
        n173 = Bundle By Name(cluster=w360, "File number counter"="Current No 2") -> (w359:T1)
        n174 = Enqueue Element(queue=w362, element="Read Data", error in (no error)=w364) -> (error out=w363:errorcluster)  [unwired: 3 out]
      }
      frame "STOP" {
        n175 = Flush Queue(queue=w373) -> (queue out=w372:refnum<queue>, error out=w371:errorcluster)  [unwired: 1 in, 1 out]
        n176 = property on="stop" class="Bool (strict)"("Val(Sgnl)"=FALSE ("Value (Signaling)")) -> ()  [unwired: 2 in, 2 out]
        n177 = Release Queue(queue=w372, error in (no error)=w371) -> (error out=w369:errorcluster)  [unwired: 3 out]
        n178 = Merge Errors(w369, w370) -> (w374:errorcluster)
      }
      frame "[Idle]" {
        n179 = Merge Errors(w377) -> (w376:errorcluster)
      }
      frame "TYPO", Default {
        n180 = Enqueue Element(queue=w384, element="STOP", error in (no error)=w383) -> (error out=w382:errorcluster)  [unwired: 3 out]
        n181 = Merge Errors(errorcluster {"status"=FALSE, "code"=0, "source"="TYPO"} ("error in 1 (no error)"), w382) -> (w381:errorcluster)
      }
    }
    "Numeric" <- w27
  }
  "error out" <- w6
